vi "SRDG535.PC Write PSDB.vi"(0 "i ref in":refnum<vi>, 5 "error IO":errorcluster) -> (14 "i ref out":refnum<vi>, 19 "error out":errorcluster)   [LabVIEW 2014, in "SRDG535.lvlib"]
doc: "This is the proc case which writes data to the PHELIX shot data base."
uses:
  SRDG535.lvlib
  CS_PHELIX/PH_Basics/PH_PSDBWriter/PH_PSDBWriter.Boolean dataset.ctl
  CS_PHELIX/PH_Basics/PH_PSDBWriter/PH_PSDBWriter.Numeric dataset.ctl
  CS_PHELIX/PH_Basics/PH_PSDBWriter/PH_PSDBWriter.String dataset.ctl
  CS_PHELIX/PH_Basics/PH_PSDBWriter/PH_PSDBWriter.lvlib
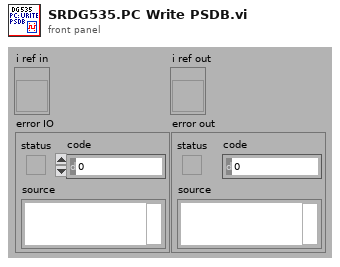
[diagram p1: front panel]
types:
  T1 = typedef "PH_PSDBWriter.lvlib/PH_PSDBWriter.String dataset.ctl" = cluster{"name":string, "data":string, "unit":string}
  T2 = typedef "PH_PSDBWriter.lvlib/PH_PSDBWriter.Numeric dataset.ctl" = cluster{"name":string, "data":dbl, "unit":string}
  T3 = typedef "PH_PSDBWriter.lvlib/PH_PSDBWriter.Boolean dataset.ctl" = cluster{"name":string, "data":bool, "unit":string}
  T4 = typedef "SRDG535.lvlib/SRDG535.i attribute.ctl" = cluster{"GPIB address":string, "Device error":errorcluster, "GUI Refs":cluster{"Delete":refnum<vi>, "Device Error":refnum<vi>, "Information":refnum<vi>, "Output":refnum<vi>, "Delay":refnum<vi>, "Trigger":refnum<vi>}, "Output Settings":T5, "Service ID Rate":i32, "Service IDs Channelinfo":i32[], "Delay Settings":T7, "Trigger Settings":T8}
  T5 = typedef "SRDG535.lvlib/SRDG535.Output.ctl" = cluster{"CH T0":T6, "CH A":T6, "CH B":T6, "CH AB":T6, "CH C":T6, "CH D":T6, "CH CD":T6}
  T6 = typedef "SRDG535.lvlib/SRDG535.Channel Output.ctl" = cluster{"Inversion":bool, "Amplitude (V)":dbl, "Offset (V)":dbl, "Mode":i32, "Load":bool}
  T7 = typedef "SRDG535.lvlib/SRDG535.Delay.ctl" = cluster{"CH A":cluster{"rel to":u32, "Delay (s)":dbl}, "CH B":cluster{"rel to":u32, "Delay (s)":dbl}, "CH C":cluster{"rel to":u32, "Delay (s)":dbl}, "CH D":cluster{"rel to":u32, "Delay (s)":dbl}}
  T8 = typedef "SRDG535.lvlib/SRDG535.Trigger.ctl" = cluster{"trigger":u32, "Impedance":bool, "Slope":bool, "burst count":i32, "external level (V)":sgl, "Internal/Burst Rate (Hz)":dbl, "Burst Period":i32}
  T9 = typedef "PH_PSDBWriter.lvlib/PH_PSDBWriter.PSDB Dataset.ctl" = cluster{"Version":i32, "2D data Input":T10[], "Boolean Input":T3[], "Image Input":T12[], "Numeric Input":T2[], "String Input":T1[]}
  T10 = typedef "PH_PSDBWriter.lvlib/PH_PSDBWriter.2D dataset.ctl" = cluster{"name":string, "data":dbl[][], "axis description":T11}
  T11 = typedef "PSDB.lvlib/PSDB_AxisDescription.ctl" = cluster{"x axis label":string, "y axis label":string, "x axis unit":string, "y axis unit":string}
  T12 = typedef "PH_PSDBWriter.lvlib/PH_PSDBWriter.Image dataset.ctl" = cluster{"name":string, "data":T13, "unit":string}
  T13 = typedef "IMAQ Image.ctl" = refnum<image>
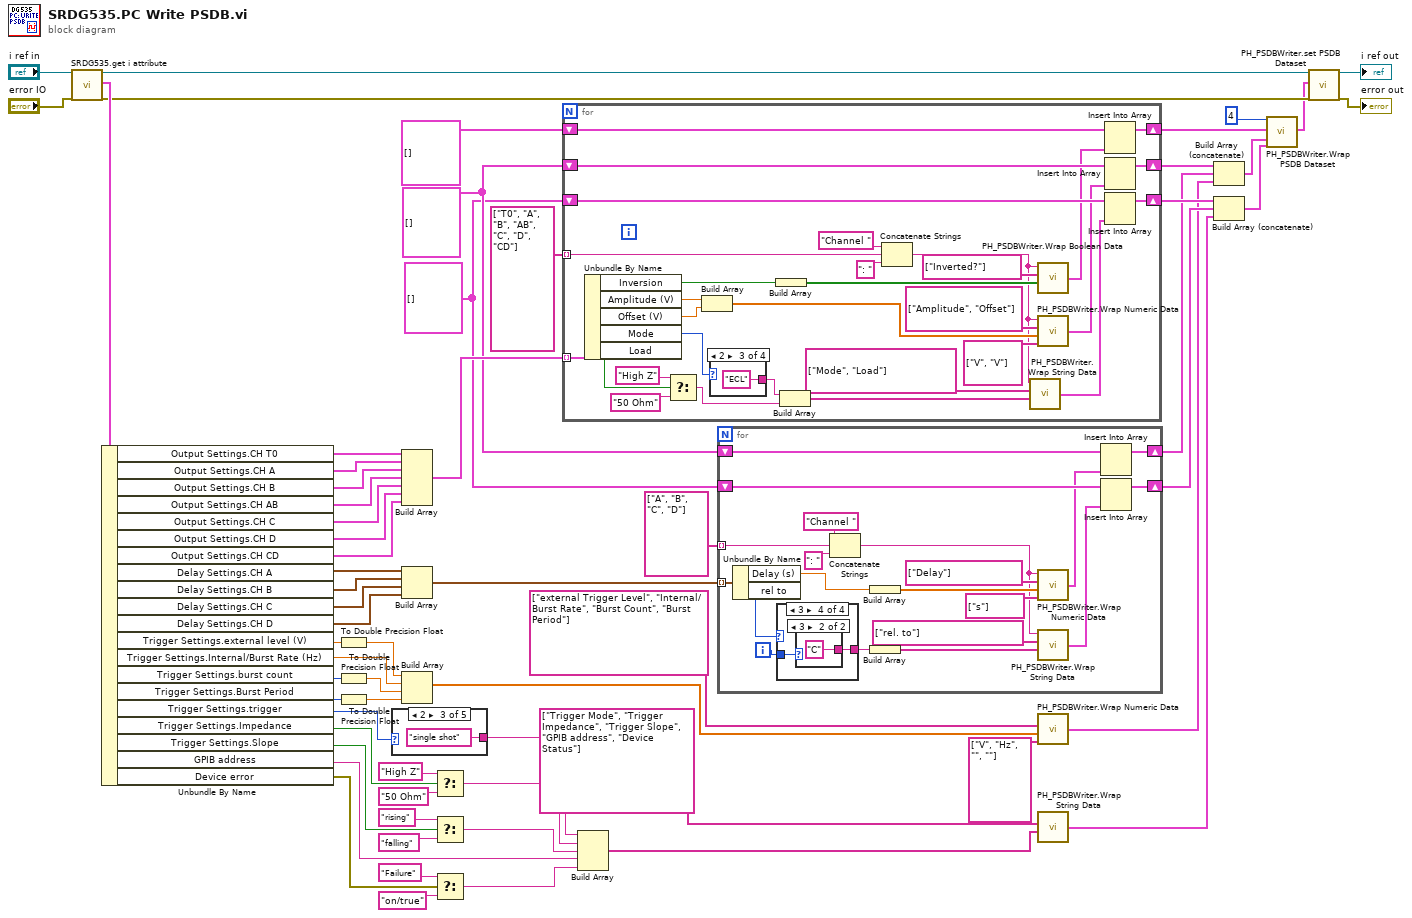
[diagram p0: block diagram]
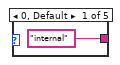
[diagram p2: hidden frame]
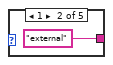
[diagram p3: hidden frame]
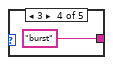
[diagram p4: hidden frame]
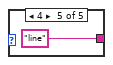
[diagram p5: hidden frame]
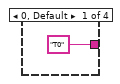
[diagram p6: hidden frame]
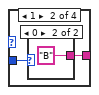
[diagram p7: hidden frame]
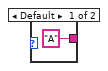
[diagram p8: hidden frame]
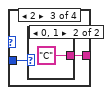
[diagram p9: hidden frame]
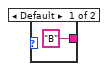
[diagram p10: hidden frame]
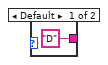
[diagram p11: hidden frame]
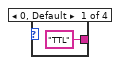
[diagram p12: hidden frame]
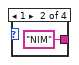
[diagram p13: hidden frame]
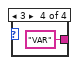
[diagram p14: hidden frame]
diagram:
  w27 = T1[] []
  w28 = T2[] []
  n1 = call "SRDG535.get i attribute.vi"("i ref in"="i ref in", "error in (no error)"="error IO") -> ("i ref out"=w18:refnum<vi>, "i attribute"=w58:T4, "error out"=w29:errorcluster)  [unwired: 15 in]
  n2 = Unbundle By Name(w58) -> ("Output Settings.CH T0"=w57:T6, "Output Settings.CH A"=w56:T6, "Output Settings.CH B"=w55:T6, "Output Settings.CH AB"=w54:T6, "Output Settings.CH C"=w53:T6, "Output Settings.CH D"=w52:T6, "Output Settings.CH CD"=w51:T6, "Delay Settings.CH A"=w49:cluster{"rel to":u32, "Delay (s)":dbl}, "Delay Settings.CH B"=w48:cluster{"rel to":u32, "Delay (s)":dbl}, "Delay Settings.CH C"=w47:cluster{"rel to":u32, "Delay (s)":dbl}, "Delay Settings.CH D"=w46:cluster{"rel to":u32, "Delay (s)":dbl}, "Trigger Settings.external level (V)"=w21:sgl, "Trigger Settings.Internal/Burst Rate (Hz)"=w44:dbl, "Trigger Settings.burst count"=w43:i32, "Trigger Settings.Burst Period"=w42:i32, "Trigger Settings.trigger"=w41:u32, "Trigger Settings.Impedance"=w38:bool, "Trigger Settings.Slope"=w36:bool, "GPIB address"=w5:string, "Device error"=w24:errorcluster)
  n3 = To Double Precision Float(number=w21) -> (double precision float=w20:dbl)
  n4 = To Double Precision Float(number=w43) -> (double precision float=w62:dbl)
  n5 = To Double Precision Float(number=w42) -> (double precision float=w61:dbl)
  n6 = case shown="2" w41 {
    tunnel: ["internal" "external" "single shot" "burst" "line"] -> w32
    frame 0, Default {
    }
    frame 1 {
    }
    frame 2 {
    }
    frame 3 {
    }
    frame 4 {
    }
  }
  n7 = Build Array(w57, w56, w55, w54, w53, w52, w51) -> (w50:T6[])
  n8 = Build Array(w49, w48, w47, w46) -> (w45:cluster{"rel to":u32, "Delay (s)":dbl}[])
  n9 = Build Array(w20, w44, w62, w61) -> (w4:dbl[])
  n10 = Select(t="High Z", s=w38, f="50 Ohm") -> (s? t:f=w33:string)
  n11 = Select(t="rising", s=w36, f="falling") -> (s? t:f=w34:string)
  n12 = Select(t="Failure", s=w24, f="on/true") -> (s? t:f=w1:string)
  n13 = for {
    tunnel: w50 -> [w98] mode=indexing
    shift-right: [w92] -> w16
    shift-left: T3[] [] -> [w91]
    shift-right: [w90] -> w60
    shift-left: w28 -> [w89]
    shift-right: [w88] -> w59
    shift-left: w27 -> [w87]
    tunnel: string[] ["T0", "A", "B", "AB", "C", "D", "CD"] -> [w80] mode=indexing
    n14 = Unbundle By Name(w98) -> ("Inversion"=w95:bool, "Amplitude (V)"=w97:dbl, "Offset (V)"=w96:dbl, "Mode"=w81:i32, "Load"=w86:bool)
    n15 = Select(t="High Z", s=w86, f="50 Ohm") -> (s? t:f=w83:string)
    n16 = Build Array(w97, w96) -> (w76:dbl[])
    n17 = case shown="2" w81 {
      tunnel: ["TTL" "NIM" "ECL" "VAR"] -> w82
      frame 0, Default {
      }
      frame 1 {
      }
      frame 2 {
      }
      frame 3 {
      }
    }
    n18 = Build Array(w95) -> (w78:bool[])
    n19 = Build Array(w82, w83) -> (w70:string[])
    n20 = Concatenate Strings("Channel ", w80, ": " ("string")) -> (w72:string)
    n21 = call "PH_PSDBWriter.Wrap String Data.vi"("Data Array"=w70, "Name Array"=string[] ["Mode", "Load"], "Name Prefix"=w72) -> ("PSDB String Data Array"=w69:T1[])  [unwired: 1 in]
    n22 = call "PH_PSDBWriter.Wrap Boolean Data.vi"("Data Array"=w78, "Name Array"=string[] ["Inverted?"], "Name Prefix"=w72) -> ("PSDB Boolean Data Array"=w77:T3[])  [unwired: 1 in]
    n23 = call "PH_PSDBWriter.Wrap Numeric Data.vi"("Unit Array"=string[] ["V", "V"], "Data Array"=w76, "Name Array"=string[] ["Amplitude", "Offset"], "Name Prefix"=w72) -> ("PSDB Numeric Data Array"=w73:T2[])
    n24 = Insert Into Array(array=w91, new element=w77) -> (w92:T3[])  [unwired: 1 in]
    n25 = Insert Into Array(array=w89, new element=w73) -> (w90:T2[])  [unwired: 1 in]
    n26 = Insert Into Array(array=w87, new element=w69) -> (w88:T1[])  [unwired: 1 in]
  }
  n27 = Build Array(w32, w33, w34, w5, w1) -> (w8:string[])
  n28 = for {
    tunnel: w45 -> [w122] mode=indexing
    shift-right: [w118] -> w26
    shift-left: w28 -> [w117]
    shift-right: [w116] -> w25
    shift-left: w27 -> [w115]
    tunnel: string[] ["A", "B", "C", "D"] -> [w111] mode=indexing
    i -> [w112]
    n29 = Unbundle By Name(w122) -> ("Delay (s)"=w121:dbl, "rel to"=w114:u32)
    n30 = case shown="3" w114 {
      tunnel: ["T0" w125 w129 w133] -> w113
      tunnel: w112 -> [_ w124 w128 w132]
      frame 0, Default {
      }
      frame 1 {
        n31 = case shown="0" w124 {
          tunnel: ["A" "B"] -> w125
          frame Default {
          }
          frame 0 {
          }
        }
      }
      frame 2 {
        n32 = case shown="0, 1" w128 {
          tunnel: ["B" "C"] -> w129
          frame Default {
          }
          frame 0, 1 {
          }
        }
      }
      frame 3 {
        n33 = case shown="3" w132 {
          tunnel: ["D" "C"] -> w133
          frame Default {
          }
          frame 3 {
          }
        }
      }
    }
    n34 = Concatenate Strings("Channel ", w111, ": " ("string")) -> (w104:string)
    n35 = Build Array(w121) -> (w107:dbl[])
    n36 = Build Array(w113) -> (w109:string[])
    n37 = call "PH_PSDBWriter.Wrap Numeric Data.vi"("Unit Array"=string[] ["s"], "Data Array"=w107, "Name Array"=string[] ["Delay"], "Name Prefix"=w104) -> ("PSDB Numeric Data Array"=w103:T2[])
    n38 = call "PH_PSDBWriter.Wrap String Data.vi"("Data Array"=w109, "Name Array"=string[] ["rel. to"], "Name Prefix"=w104) -> ("PSDB String Data Array"=w108:T1[])  [unwired: 1 in]
    n39 = Insert Into Array(array=w117, new element=w103) -> (w118:T2[])  [unwired: 1 in]
    n40 = Insert Into Array(array=w115, new element=w108) -> (w116:T1[])  [unwired: 1 in]
  }
  n41 = call "PH_PSDBWriter.Wrap Numeric Data.vi"("Unit Array"=string[] ["V", "Hz", "", ""], "Data Array"=w4, "Name Array"=string[] ["external Trigger Level", "Internal/Burst Rate", "Burst Count", "Burst Period"]) -> ("PSDB Numeric Data Array"=w9:T2[])  [unwired: 1 in]
  n42 = call "PH_PSDBWriter.Wrap String Data.vi"("Data Array"=w8, "Name Array"=string[] ["Trigger Mode", "Trigger Impedance", "Trigger Slope", "GPIB address", "Device Status"]) -> ("PSDB String Data Array"=w6:T1[])  [unwired: 2 in]
  n43 = Build Array (concatenate)(w60, w26, w9) -> (w15:T2[])
  n44 = Build Array (concatenate)(w59, w25, w6) -> (w14:T1[])
  n45 = call "PH_PSDBWriter.Wrap PSDB Dataset.vi"("Version"=4, "Boolean Input"=w16, "Numeric Input"=w15, "String Input"=w14) -> ("PSDB Dataset"=w12:T9)  [unwired: 15 in]
  n46 = call "PH_PSDBWriter.set PSDB Dataset.vi"("VI in"=w18, "PSDB Dataset"=w12, "error in (no error)"=w29) -> ("VI out"=→"i ref out":refnum<vi>, "error out"=→"error out":errorcluster)  [unwired: 15 in]
